vi "Commmand.vi"(7 "Param 2":string, 9 "Param1":string, 10 "Command":T1, 11 "Serial Device Brand":T2) -> (3 "Command to send":string)   [LabVIEW 2020, in "Serial Device.lvclass"]
uses:
  Serial Device.lvclass
  implementations/Combo box/serial device brand.ctl
  command.ctl
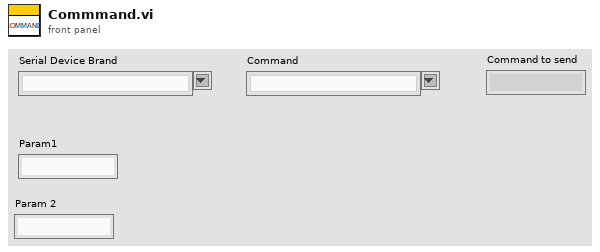
[diagram p1: front panel]
types:
  T1 = typedef "Serial Device.lvclass/command.ctl" = string
  T2 = typedef "Serial Device.lvclass/serial device brand.ctl" = string
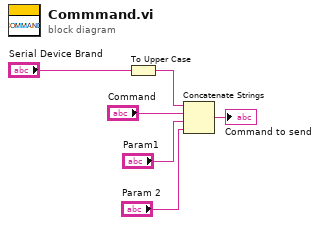
[diagram p0: block diagram]
diagram:
  n1 = To Upper Case(1:"Serial Device Brand") -> (0:w4:T2)
  n2 = Concatenate Strings(w4, "Command", "Param1", "Param 2") -> (→"Command to send":string)
